vi "Pulsed Experiment - memory leak bug.vi"(0 "Optimize Parameters":T3={"Volt Step"={"X"=0.01, "Y"=0.01, "Z"=0.0}, "Num Iterations"=1, "Dwell Time (ms)"=100, "Volts Range"={"X"=0.1, "Y"=0.1, "Z"=0.0}, "Method"={"X"=enum."Max", "Y"=enum."Max", "Z"=enum."Max"}} {"Volts Range"."Z" min=0.0; "Volts Range"."Y" min=0.0; "Volts Range"."X" min=0.0; "Dwell Time (ms)" min=0; "Num Iterations" min=1 step=1; "Volt Step"."Z" min=1e-05; "Volt Step"."Y" min=1e-06; "Volt Step"."X" min=1e-06}, 3 "Contrast XY Graph Refnum":refnum<vi>, 4 "Experiment":T1=enum."Rabi", 5 "# samples":i32, 7 "# time points":i32, 9 "min time":dbl, 11 "max time":dbl, 12 "# scan iterations":i32, 13 "Window Parameters":string, 14 "Save Contrast Options":T2={"Save contrast graph"=FALSE, "Path for contrast graph"=path "C:/experiment/data/may_15_2012/SIL1_NV1_pippin_uW_off", "Save contrast data"=FALSE, "Path for contrast data"=path "C:/experiment/data/may_15_2012/SIL1_NV1_pippin_uW_off"}, 15 "scans done ref":refnum<vi>) -> ()   [LabVIEW 2012]
uses:
  Strict Type Def - Optimize Parameters Cluster.ctl
  SaveContrastOptions.ctl
  States.ctl
  <vilib>/DAQmx/read.llb/DAQmx Read (Counter 1D U32 1Chan NSamp).vi
  Channels.vi
  <vilib>/DAQmx/miscellaneous.llb/DAQmx Fill In Error Info.vi
  Global Vars.vi
  <vilib>/Analysis/baseanly.llb/Mean (DBL).vi
  <vilib>/Utility/file.llb/Write To Spreadsheet File (DBL).vi
  <vilib>/Analysis/NI_AALBase.lvlib
panel:
  in  "tracking counts ref":refnum<vi>
  out "Counts/s":u32
  out "scans done":u32
  out "Readout counts":cluster{"Y":dbl[], "Y":dbl[]}[](graph)
  out "Reference counts":cluster{"Y":dbl[], "Y":dbl[]}[](graph)
  out "Normalized contrast":cluster{"Y":dbl[], "Y":dbl[]}[](graph)
  # "Pulsed Experiments: \nData collection and processing\nRabi\nSpin Echo\nCPMG\nXY-4\n\n08/27/2013, Srujan Meesala\n6/9/2014, Samuel Kim"
  # "Default PB connections:\nPB0 - MW switch\nPB1 - unused\nPB2 - Counter sample clk\nPB3 - Green AOM"
  # "Pulse sequence parameters"
  # "to spreadsheet"
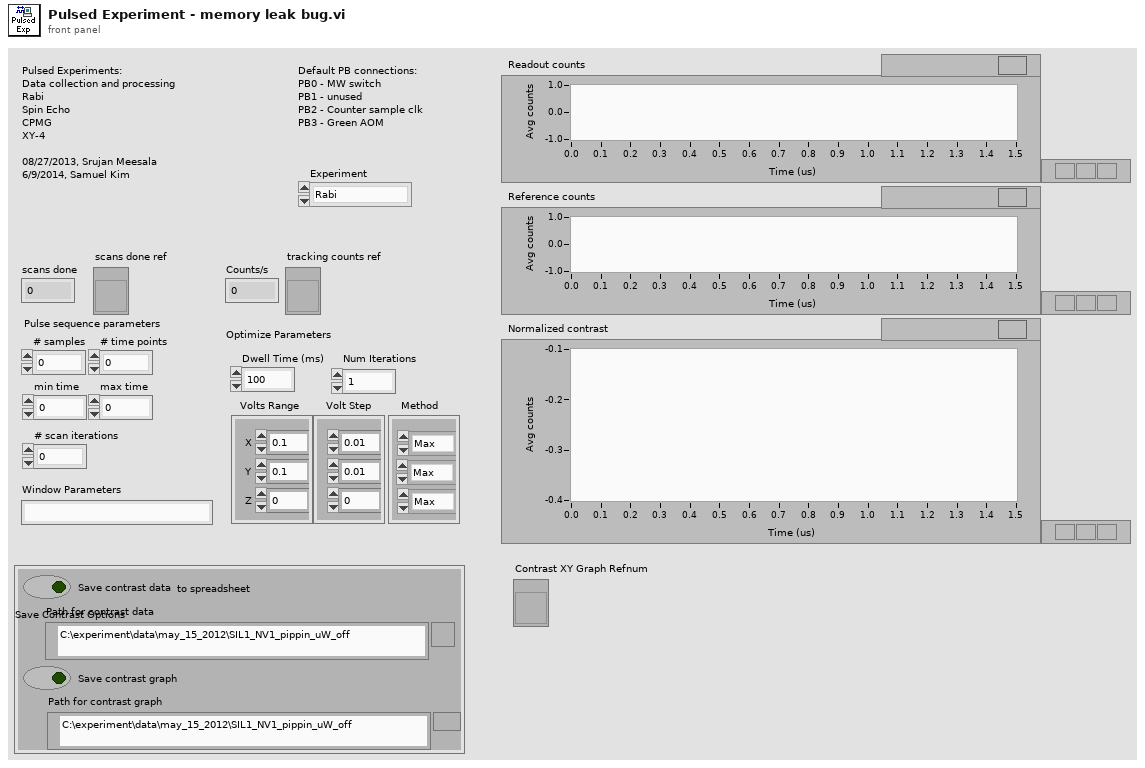
[diagram p1: front panel]
types:
  T1 = typedef "States.ctl" = enum16{"Initialize", "Scan", "Count", "Optimize", "Hold", "ESR", "Rabi", "Spin Echo", "Spectrum", "Stability", "CPMG", "XY-4", "Exit"}
  T2 = typedef "SaveContrastOptions.ctl" = cluster{"Save contrast graph":bool, "Path for contrast graph":path, "Save contrast data":bool, "Path for contrast data":path}
  T3 = typedef "Strict Type Def - Optimize Parameters Cluster.ctl" = cluster{"Volt Step":cluster{"X":dbl, "Y":dbl, "Z":dbl}, "Num Iterations":i32, "Dwell Time (ms)":i32, "Volts Range":cluster{"X":dbl, "Y":dbl, "Z":dbl}, "Method":cluster{"X":enum16{"Max", "Gaussian"}, "Y":enum16{"Max", "Gaussian"}, "Z":enum16{"Max", "Gaussian"}}}
  T4 = typedef "imagedata.ctl" = cluster{"image type":i32, "image depth":i32, "image":u8[], "mask":u8[], "colors":u32[], "Rectangle":cluster{"left":i16, "top":i16, "right":i16, "bottom":i16}}
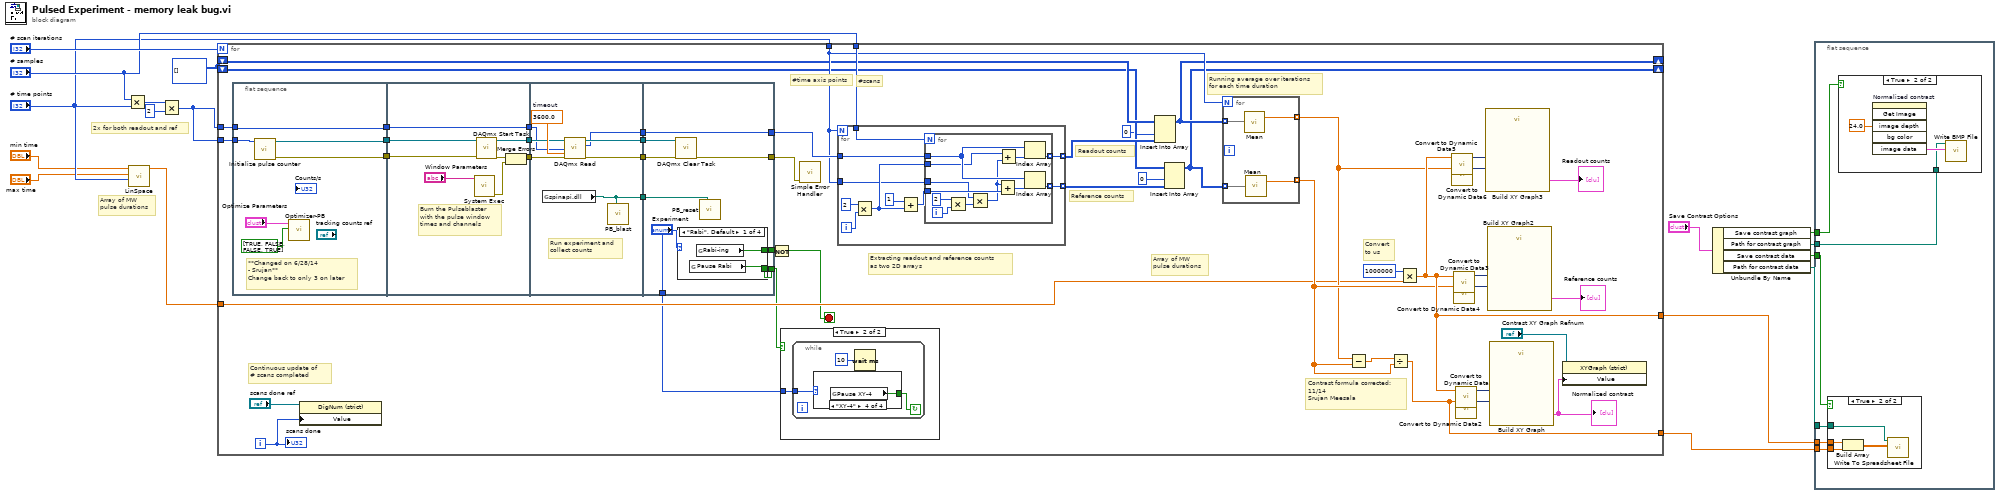
[diagram p0: block diagram]
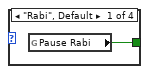
[diagram p5: hidden frame]
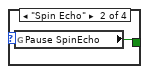
[diagram p6: hidden frame]
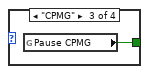
[diagram p7: hidden frame]
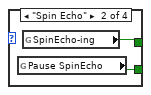
[diagram p8: hidden frame]
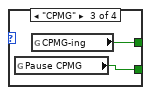
[diagram p9: hidden frame]
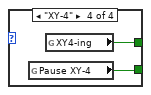
[diagram p10: hidden frame]
diagram:
  w12 = i32[][] [] ("Flourescence Data")
  # "Array of MW\npulse durations"
  # "2x for both readout and ref"
  n1 = Multiply(x="# samples", y="# time points") -> (x*y=w15:i32)
  n2 = call "LinSpace.vi"("Num Steps"="# time points", "Max"="max time", "Min"="min time") -> ("Array"=w10:dbl[])  [unwired: 8 in]
  n3 = Multiply(x=w15, y=u32 2 ("Reset Count")) -> (x*y=w13:u32)
  n4 = for {
    N: "# scan iterations" -> [_]
    tunnel: [w48] -> w17
    tunnel: [w46] -> w16
    tunnel: w13 -> [w44]
    tunnel: "# samples" -> [w43]
    tunnel: "# time points" -> [w42]
    tunnel: w13 -> [w41]
    shift-right: [w36] -> _
    shift-left: w12 -> [w37]
    shift-right: [w28] -> _
    shift-left: w12 -> [w34]
    tunnel: w10 -> [w25]
    i -> [w18]
    stop <- w22 stop-if-true
    # "Continuous update of \n# scans completed"
    # "Convert\nto us"
    # "Contrast formula corrected:\n11/14\nSrujan Meesala"
    # "#time axis points"
    # "#scans"
    # "Reference counts"
    # "Readout counts"
    # "Running average over iterations\nfor each time duration"
    # "Array of MW\npulse durations"
    # "Extracting readout and reference counts\nas two 2D arrays"
    n5 = flat-sequence {
      tunnel: w44 -> [w78]
      tunnel: [w78] -> w64
      tunnel: w41 -> [w76]
      tunnel: [w75] -> w40
      tunnel: [w74] -> w39
      tunnel: [w86] -> w63
      tunnel: [w85] -> w62
      tunnel: w64 -> [w85]
      tunnel: w40 -> [w84]
      tunnel: w39 -> [w83]
      tunnel: [w80] -> w24
      tunnel: w63 -> [w93]
      tunnel: [w89] -> w61
      tunnel: [w91] -> w60
      tunnel: [w90] -> w59
      tunnel: w62 -> [w88]
      tunnel: [w87] -> w58
      tunnel: w24 -> [w92]
      tunnel: [w102] -> w56
      tunnel: w61 -> [w102]
      tunnel: w60 -> [w101]
      tunnel: w59 -> [w99]
      tunnel: [w98] -> w57
      tunnel: w58 -> [w100]
      tunnel: [w97] -> w23
      tunnel: [w96] -> w21
      tunnel: ["Experiment"] -> w20
      frame #0 {
        # "**Changed on 6/28/14\n- Srujan**\nChange back to only 3 on later"
        n6 = call "Initialize pulse counter.vi"("Samples per channel"=w76) -> ("error out"=w74:errorcluster, "DAQmx Task Name"=w75:refnum<k21>)  [unwired: 9 in]
        n7 = call "Optimizer-PB.vi"("Optimize active channels"=bool[] [TRUE, FALSE, FALSE, TRUE], "Optimize Parameters"="Optimize Parameters") -> ()  [unwired: 9 in, 1 out]
      }
      frame #1 {
        # "Burn the Pulseblaster\nwith the pulse window\ntimes and channels"
        n8 = call <vilib>:"System Exec.vi"("command line"="Window Parameters") -> ("error out"=w82:errorcluster)  [unwired: 7 in, 3 out]
        n9 = call <vilib>:"DAQmx Start Task.vi"("task/channels in"=w84, "error in"=w83) -> ("task out"=w86:refnum<k21>, "error out"=w81:errorcluster)  [unwired: 12 in]
        n10 = Merge Errors(w81, w82) -> (w80:errorcluster)
      }
      frame #2 {
        w94 = 3600.0  # timeout
        # "Run experiment and\ncollect counts"
        n11 = global read "Channels.vi" "spinapi.dll"() -> (w87:path)
        n12 = call-poly <vilib>:"DAQmx Read.vi"("task/channels in"=w93, "number of samples per channel"=w88, "timeout"=w94, "error in"=w92) -> ("task out"=w90:refnum<k21>, "data"=w89:u32[], "error out"=w91:errorcluster)  [unwired: 9 in]
        n13 = call "PB_blast.vi"("Path to spinapi.dll"=w87) -> ()  [unwired: 7 in]
      }
      frame #3 {
        n14 = call <vilib>:"DAQmx Clear Task.vi"("task in"=w99, "error in"=w101) -> ("error out"=w98:errorcluster)  [unwired: 13 in]
        n15 = case shown="\"Rabi\", Default" "Experiment" {
          tunnel: [w104 w106 w108 w110] -> w97
          tunnel: [w103 w105 w107 w109] -> w96
          frame "Rabi", Default {
            n16 = global read "Global Vars.vi" "Pause Rabi"() -> (w103:bool)
            n17 = global read "Global Vars.vi" "Rabi-ing"() -> (w104:bool)
          }
          frame "Spin Echo" {
            n18 = global read "Global Vars.vi" "Pause SpinEcho"() -> (w105:bool)
            n19 = global read "Global Vars.vi" "SpinEcho-ing"() -> (w106:bool)
          }
          frame "CPMG" {
            n20 = global read "Global Vars.vi" "Pause CPMG"() -> (w107:bool)
            n21 = global read "Global Vars.vi" "CPMG-ing"() -> (w108:bool)
          }
          frame "XY-4" {
            n22 = global read "Global Vars.vi" "Pause XY-4"() -> (w109:bool)
            n23 = global read "Global Vars.vi" "XY4-ing"() -> (w110:bool)
          }
        }
        n24 = call "PB_reset.vi"("Path to spinapi.dll"=w100) -> ()  [unwired: 7 in]
      }
    }
    n25 = property class="DigNum (strict)"(reference="scans done ref", "Value"=w18) -> ()  [unwired: 1 in, 2 out]
    n26 = Not(x=w23) -> (.not. x?=w22:bool)
    n27 = case shown="True" w21 {
      tunnel: w20 -> [_ w65]
      frame False {
      }
      frame True {
        n28 = while {
          tunnel: w65 -> [w66]
          stop <- w67 continue-if-true
          n29 = case shown="\"XY-4\"" w66 {
            tunnel: [w69 w70 w71 w72] -> w67
            frame "Rabi", Default {
              n30 = global read "Global Vars.vi" "Pause Rabi"() -> (w69:bool)
            }
            frame "Spin Echo" {
              n31 = global read "Global Vars.vi" "Pause SpinEcho"() -> (w70:bool)
            }
            frame "CPMG" {
              n32 = global read "Global Vars.vi" "Pause CPMG"() -> (w71:bool)
            }
            frame "XY-4" {
              n33 = global read "Global Vars.vi" "Pause XY-4"() -> (w72:bool)
            }
          }
          n34 = Wait (ms)(milliseconds to wait=u32 10) -> ()  [unwired: 1 out]
        }
      }
    }
    n35 = call <vilib>:"Simple Error Handler.vi"("error in (no error)"=w57) -> ()  [unwired: 4 in, 5 out]
    n36 = for {
      N: w42 -> [_]
      tunnel: w43 -> [w123]
      tunnel: w56 -> [w124]
      tunnel: [w122] -> w38 mode=indexing
      tunnel: [w121] -> w35 mode=indexing
      tunnel: w42 -> [w115]
      i -> [w120]
      n37 = Multiply(x=u32 2 ("Reset Count"), y=w120) -> (x*y=w117:u32)
      n38 = Add(x=u32 1 ("Reset Count"), y=w117) -> (x+y=w116:u32)
      n39 = for {
        N: w123 -> [_]
        tunnel: w124 -> [w136]
        tunnel: [w133] -> w122 mode=indexing
        tunnel: [w132] -> w121 mode=indexing
        tunnel: w117 -> [w131]
        tunnel: w116 -> [w130]
        tunnel: w115 -> [w126]
        i -> [w128]
        n40 = Multiply(x=u32 2 ("Reset Count"), y=w128) -> (x*y=w127:u32)
        n41 = Multiply(x=w126, y=w127) -> (x*y=w125:u32)
        n42 = Add(x=w125, y=w130) -> (x+y=w134:u32)
        n43 = Add(x=w131, y=w125) -> (x+y=w135:u32)
        n44 = Index Array(array=w136, index=w135) -> (element=w133:u32)
        n45 = Index Array(array=w136, index=w134) -> (element=w132:u32)
      }
    }
    n46 = Insert Into Array(array=w37, index (col)=u32 0 ("Reset Count"), new element=w38) -> (w36:i32[][])  [unwired: 1 in]
    n47 = Insert Into Array(array=w34, index (col)=u32 0 ("Reset Count"), new element=w35) -> (w28:i32[][])  [unwired: 1 in]
    n48 = for {
      N: w42 -> [_]
      tunnel: w36 -> [w114] mode=indexing
      tunnel: w28 -> [w113] mode=indexing
      tunnel: [w112] -> w45 mode=indexing
      tunnel: [w111] -> w29 mode=indexing
      n49 = call-poly <vilib>:"Mean.vi"("X"=w114) -> ("mean"=w111:dbl)  [unwired: 1 out]
      n50 = call-poly <vilib>:"Mean.vi"("X"=w113) -> ("mean"=w112:dbl)  [unwired: 1 out]
    }
    n51 = Subtract(x=w29, y=w45) -> (x-y=w47:dbl[])
    n52 = Divide(x=w47, y=w45) -> (x/y=w48:dbl[])
    n53 = Multiply(x=u32 1000000 ("Reset Count"), y=w25) -> (x*y=w46:dbl[])
    n54 = call "Convert to Dynamic Data5"("Array"=w46) -> ("Dynamic Data Type"=w50:dynamicdata)  [unwired: 3 in]
    n55 = call "Convert to Dynamic Data6"("Array"=w29) -> ("Dynamic Data Type"=w49:dynamicdata)  [unwired: 3 in]
    n56 = call "Convert to Dynamic Data3"("Array"=w46) -> ("Dynamic Data Type"=w53:dynamicdata)  [unwired: 3 in]
    n57 = call "Convert to Dynamic Data4"("Array"=w45) -> ("Dynamic Data Type"=w52:dynamicdata)  [unwired: 3 in]
    n58 = call "Convert to Dynamic Data"("Array"=w46) -> ("Dynamic Data Type"=w55:dynamicdata)  [unwired: 3 in]
    n59 = call "Convert to Dynamic Data2"("Array"=w48) -> ("Dynamic Data Type"=w54:dynamicdata)  [unwired: 3 in]
    n60 = call "Build XY Graph3"("Y Input"=w49, "X Input"=w50) -> ("XY Graph"=→"Readout counts":cluster{"Y":dbl[], "Y":dbl[]}[])  [unwired: 3 in, 6 out]
    n61 = call "Build XY Graph2"("Y Input"=w52, "X Input"=w53) -> ("XY Graph"=→"Reference counts":cluster{"Y":dbl[], "Y":dbl[]}[])  [unwired: 3 in, 6 out]
    n62 = call "Build XY Graph"("Y Input"=w54, "X Input"=w55) -> ("XY Graph"=w30:cluster{"Y":dbl[], "Y":dbl[]}[])  [unwired: 3 in, 6 out]
    "Normalized contrast" <- w30
    n63 = property class="XYGraph (strict)"(reference="Contrast XY Graph Refnum", "Value"=w30) -> ()  [unwired: 1 in, 2 out]
    "scans done" <- w18
  }
  n64 = Unbundle By Name("Save Contrast Options") -> ("Save contrast graph"=w4:bool, "Path for contrast graph"=w2:path, "Save contrast data"=w3:bool, "Path for contrast data"=w1:path)
  n65 = flat-sequence {
    tunnel: w17 -> [w142]
    tunnel: w16 -> [w141]
    tunnel: w4 -> [w140]
    tunnel: w3 -> [w139]
    tunnel: w2 -> [w138]
    tunnel: w1 -> [w137]
    frame #0 {
      n66 = case shown="True" w139 {
        tunnel: w141 -> [_ w144]
        tunnel: w142 -> [_ w145]
        tunnel: w137 -> [_ w143]
        frame False {
        }
        frame True {
          n67 = Build Array(w144, w145) -> (w146:dbl[][])
          n68 = call-poly <vilib>:"Write To Spreadsheet File.vi"("2D data"=w146, "file path (dialog if empty)"=w143) -> ()  [unwired: 6 in, 1 out]
        }
      }
      n69 = case shown="True" w140 {
        tunnel: w138 -> [_ w147]
        frame False {
        }
        frame True {
          n70 = invoke on="Normalized contrast" class="XYGraph (strict)" method="Get Image"("image depth"=24.0 ("Initial Delay")) -> ("image data"=w148:T4)  [unwired: 5 in, 5 out]
          n71 = call <vilib>:"Write BMP File.vi"("image data"=w148, "path to BMP file"=w147) -> ()  [unwired: 8 in, 2 out]
        }
      }
    }
  }
